vi "四分频(T'触发器).vi"(2 "error in (no error)":errorcluster caption="错误输入（无错误）", 3 "CP":bool) -> (0 "error out":errorcluster caption="错误输出", 1 "Q":bool)   [LabVIEW 2012, in "触发器.lvlib"]
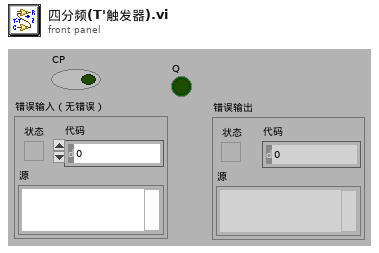
[diagram p1: front panel]
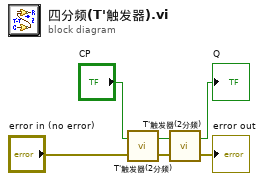
[diagram p0: block diagram]
diagram:
  n1 = call "T'触发器(2分频).vi"("error in (no error)"="error in (no error)", "CP"="CP") -> ("error out"=w1:errorcluster, "Q"=w5:bool)
  n2 = call "T'触发器(2分频).vi"("error in (no error)"=w1, "CP"=w5) -> ("error out"=→"error out":errorcluster, "Q"=→"Q":bool)
